vi "Zstack Save Image.vi"(8 "error in (no error)":errorcluster, 9 "Dataset base-path":path, 11 "Image Array":T1) -> (0 "error out":errorcluster)   [LabVIEW 2017]
uses:
  User Interface/Queue/Live graphs queue/Typedefs/Live imaging queue element.ctl
  <vilib>/vision/Image Controls.llb/IMAQ Image.ctl
  <vilib>/vision/NI_Vision_Development_Module.lvlib
panel:
  out "Array":path[](array[path])
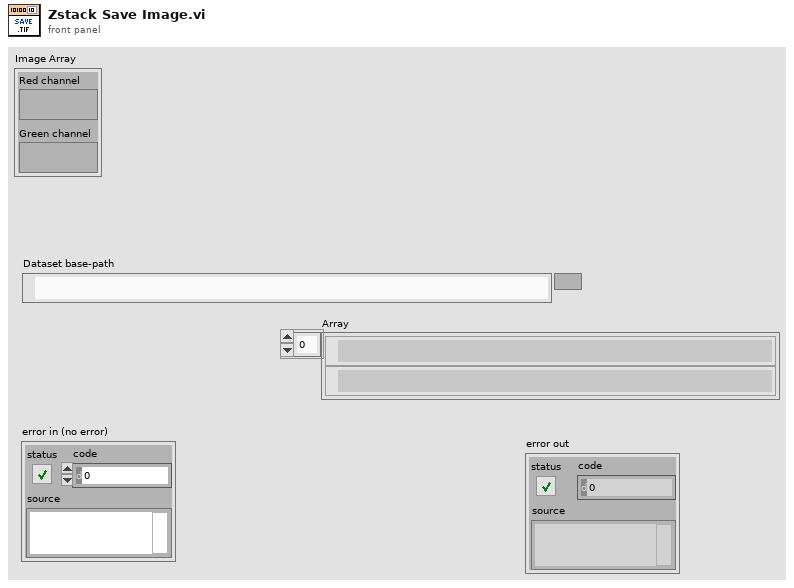
[diagram p1: front panel]
types:
  T1 = typedef "Live imaging queue element.ctl" = cluster{"Red channel":T2, "Green channel":T2}
  T2 = typedef "IMAQ Image.ctl" = refnum<image>
  T3 = typedef "Fixed strings.ctl" = cluster{"ROI file name":string, "Normalised ROI file name":string, "Zplane Pockels values file name":string, "Functional data folder name":string, "Experiment Header file name":string, "Z-stack images folder name":string, "Groups setup rel. path":string, "Groups text file rel. path":string, "TDMS files folder name (F.img)":string, "TDMS files folder name (V.acq)":string, "TDMS files folder name (Pl.acq)":string, "Cycle rel times sequence file":string, "Dynamically called VIs folder name":string, "Time Series folder base name":string}
  T4 = cluster{"Rows Per Strip":i32, "Photometric":i32, "Compression Type":i32}
  T5 = typedef "Image Type" = u32
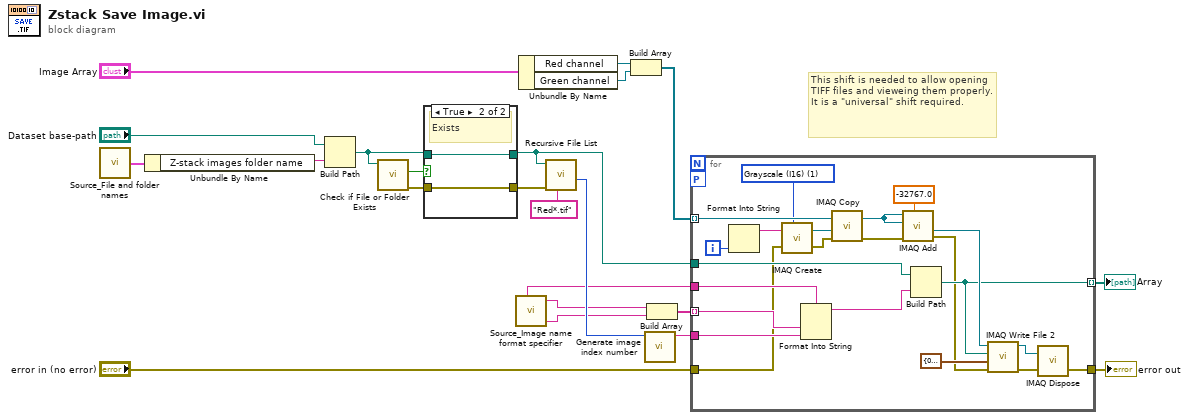
[diagram p0: block diagram]
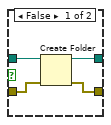
[diagram p2: hidden frame]
diagram:
  # "This shift is needed to allow opening TIFF files and vieweing them properly.\nIt is a \"universal\" shift required."
  n1 = call "Source_File and folder names.vi"() -> ("Fixed strings"=w8:T3)  [unwired: 1 in]
  n2 = Unbundle By Name(w8) -> ("Z-stack images folder name"=w7:string)
  n3 = Build Path(base path="Dataset base-path", name or relative path=w7) -> (appended path=w17:path)
  n4 = call <vilib>:"Check if File or Folder Exists.vi"("path"=w17) -> ("error out"=w15:errorcluster, "file or folder exists?"=w16:bool)  [unwired: 8 in, 1 out]
  n5 = case shown="True" w16 {
    tunnel: [w26 w27] -> w18
    tunnel: w17 -> [w25 w27]
    tunnel: w15 -> [w24 w28]
    tunnel: [w23 w28] -> w14
    frame False {
      n6 = Create Folder(path (use dialog)=w25, error in=w24) -> (created path=w26:path, error out=w23:errorcluster)  [unwired: 1 in, 1 out]
    }
    frame True {
      # "Exists"
    }
  }
  n7 = call "Source_Image name format specifier.vi"() -> ("Z-Stack Image name format specifier"=w10:string, "Red channel name"=w6:string, "Green channel name"=w5:string)  [unwired: 5 in]
  n8 = Unbundle By Name("Image Array") -> ("Red channel"=w2:T2, "Green channel"=w3:T2)
  n9 = call <vilib>:"Recursive File List.vi"("pattern"="Red*.tif", "error in (no error)"=w14, "Folder Path"=w18) -> ("Number of Files"=w13:i32)  [unwired: 4 in, 4 out]
  n10 = Build Array(w2, w3) -> (w1:T2[])
  n11 = call "Generate image index number.vi"("FOR loop iteration or existing number of files"=w13) -> ("Number in string representation (padded with zeroes)"=w12:string)  [unwired: 10 in]
  n12 = Build Array(w6, w5) -> (w9:string[])
  n13 = for {
    tunnel: w18 -> [w50]
    tunnel: w9 -> [w48] mode=indexing
    workers-P: _ -> [_]
    tunnel: "error in (no error)" -> [w37]
    tunnel: [w33] -> w20
    tunnel: w12 -> [w47]
    tunnel: [w45] -> w11 mode=indexing
    tunnel: w10 -> [w44]
    tunnel: w1 -> [w35] mode=indexing
    i -> [w30]
    w29 = T5 1 items=["Grayscale (U8)", "Grayscale (I16)", "Grayscale (SGL)", "Complex (CSG)", "RGB (U32)", "HSL (U32)", "RGB (U64)", "Grayscale (U16)"] ("Image Type")
    n14 = Format Into String(w30) -> (resulting string=w31:string)  [unwired: 3 in, 1 out]
    n15 = call "IMAQ Create"("Image Name"=w31, "Image Type"=w29, "error in (no error)"=w37) -> ("New Image"=w41:T2, "error out"=w39:errorcluster)  [unwired: 2 in]
    n16 = Format Into String(format string=w44, w48, w47) -> (resulting string=w46:string)  [unwired: 2 in, 1 out]
    n17 = call "IMAQ Copy"("error in (no error)"=w39, "Image Dst"=w41, "Image Src"=w35) -> ("error out"=w38:errorcluster, "Image Dst Out"=w40:T2)  [unwired: 3 in]
    n18 = call "IMAQ Add"("Image Src A"=w40, "Constant"=-32767.0, "Image Dst"=w40, "error in (no error)"=w38) -> ("Image Dst Out"=w49:T2, "error out"=w36:errorcluster)  [unwired: 3 in]
    n19 = Build Path(base path=w50, name or relative path=w46) -> (appended path=w45:path)
    n20 = call-poly "IMAQ Write File 2"("error in (no error)"=w36, "TIFF Options"=T4 {"Rows Per Strip"=0, "Photometric"=1, "Compression Type"=0}, "File Path"=w45, "Image"=w49) -> ("error out"=w34:errorcluster, "Image Out (duplicate)"=w32:T2)  [unwired: 6 in]
    n21 = call "IMAQ Dispose"("Image"=w32, "error in (no error)"=w34) -> ("error out"=w33:errorcluster)  [unwired: 4 in]
  }
  "error out" <- w20
  "Array" <- w11
